vi "Z6_Beamline_Chief.ProcCases.vi"(0 "i ref in":refnum<vi>, 1 "selector":string, 2 "Data":T1, 3 "call cluster":T2={"Object"="", "Selector"="", "CallType"=enum."synchronous", "Async Object"="", "Async Selector"="", "Data Descriptor"="", "Data"=[], "Error #"=0, "Expire"=0}, 5 "error in (no error)":errorcluster) -> (14 "i ref out":refnum<vi>, 17 "answer cluster":T2={"Object"="", "Selector"="", "CallType"=enum."synchronous", "Async Object"="", "Async Selector"="", "Data Descriptor"="", "Data"=[], "Error #"=0, "Expire"=0}, 19 "error out":errorcluster)   [LabVIEW 2014, in "Z6_Beamline_Chief.lvlib"]
doc: "This method is called by a process from within the default case in the event loop. The methods of a class that are linked to events will be called from THIS method. Add your code here."
uses:
  Z6_Beamline_Chief.lvlib
  CSCore/CSSystem/CoreDefs/CoreDefs.call_type.ctl
  CSCore/BaseProcess/BaseProcess.descriptor string definition.ctl
  CSCore/CSSystem/CoreDefs/CoreDefs.rawDataType.ctl
  PH_BL-Master/PH_BL-Master.lvlib
  Z6_Beamline/Z6_Beamline.lvlib
  CSCore/BaseProcess/BaseProcess.lvlib
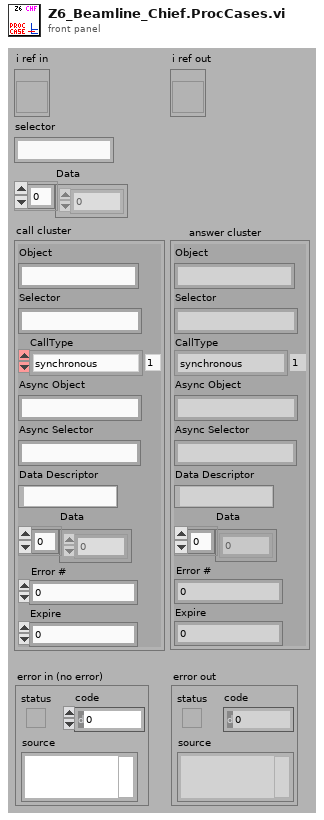
[diagram p1: front panel]
types:
  T1 = typedef "CoreDefs.rawDataType.ctl" = i8[]
  T2 = typedef "CoreDefs.call_type.ctl" = cluster{"Object":string, "Selector":string, "CallType":enum16{"simple", "synchronous", "asynchronous"}, "Async Object":string, "Async Selector":string, "Data Descriptor":T3, "Data":T1, "Error #":i32, "Expire":u32}
  T3 = typedef "BaseProcess.lvlib/BaseProcess.descriptor string definition.ctl" = string
  T4 = typedef "PH_BL-Master.lvlib/PH_BL-Master.i attribute.ctl" = cluster{"Remote controlled":bool, "Boolean Condition Service Subscriber":refnum<vi>[], "Picture Condition Service Subscriber":refnum<vi>[], "R2S":cluster{"GUI Ref":refnum<vi>, "State":bool}, "Vacua":cluster{"GUI Ref":refnum<vi>, "Limit":dbl, "Curr Value":dbl, "in range":bool}[], "O2 Inspection":cluster{"GUI Ref":refnum<vi>, "Concentration":dbl, "State":T5}[], "Boolean Status Service Subscriber":cluster{"GUI Ref":refnum<vi>, "Status":T5, "no Link?":bool, "Status Subscriber Class":T6}[], "Picture Status Service Subscriber":cluster{"GUI Ref":refnum<vi>, "Status":T5, "no Link?":bool, "Status Subscriber Class":T6}[], "6P 4Q Service Subscriber":cluster{"GUI Ref":refnum<vi>, "Selector":T7, "no Link?":bool}[], "Index of latest 6P 4Q changing Instance":i32, "Index of latest Picture Status changing Instance":i32, "Index of latest Boolean Status changing Instance":i32, "Vision ID on same Node":string, "Start Phase over?":bool, "GUI Ref Delete":refnum<vi>}
  T5 = typedef "PH_StatusHandler.lvlib/PH_StatusHandler.Status.ctl" = i16
  T6 = typedef "PH_BL-Master.lvlib/PH_BL-Master.Status Subscriber Class.ctl" = enum16{"unknown", "Switch", "BB", "6P Switch", "Switch GUI", "Switch and 6P State", "Force Sensor"}
  T7 = typedef "PH_4_Pos_Selector.lvlib/PH_4_Pos_Selector.Position Selector.ctl" = u16
  T8 = cluster{"GUI Ref":refnum<vi>, "Status":T5, "no Link?":bool, "Status Subscriber Class":T6}[]
  T9 = cluster{"GUI Ref":refnum<vi>, "Limit":dbl, "Curr Value":dbl, "in range":bool}[]
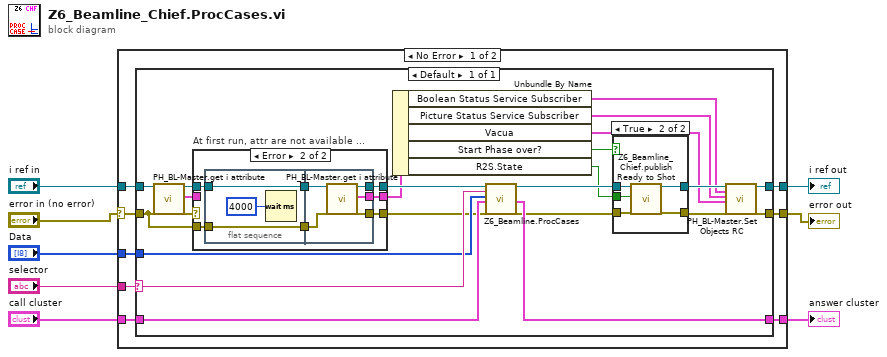
[diagram p0: block diagram]
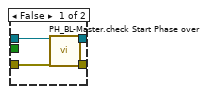
[diagram p3: hidden frame]
diagram:
  n1 = case shown="No Error" "error in (no error)" {
    selector: "error in (no error)" -> [w9 w68]
    tunnel: "selector" -> [w16 _]
    tunnel: [w15 w67] -> w7
    tunnel: "call cluster" -> [w14 w67]
    tunnel: "i ref in" -> [w13 w69]
    tunnel: [w12 w69] -> w4
    tunnel: [w11 w68] -> w3
    tunnel: "Data" -> [w10 _]
    frame No Error {
      n2 = case shown="Default" w16 {
        selector: w16 -> [w37]
        tunnel: w13 -> [w22]
        tunnel: [w33] -> w12
        tunnel: w14 -> [w38]
        tunnel: [w39] -> w15
        tunnel: w9 -> [w20]
        tunnel: [w32] -> w11
        tunnel: w10 -> [w36]
        frame Default {
          n3 = call "PH_BL-Master.get i attribute.vi"("i ref in"=w22, "error in (no error)"=w20) -> ("i ref out"=w21:refnum<vi>, "i attribute"=w18:T4, "error out"=w19:errorcluster)  [unwired: 15 in]
          n4 = case "At first run, attr are not available ..." shown="Error" w19 {
            selector: w19 -> [w41 _]
            tunnel: [w41 w49] -> w31
            tunnel: [w42 w48] -> w30
            tunnel: [w40 w47] -> w27
            tunnel: w21 -> [w42 w46]
            tunnel: w20 -> [_ w45]
            tunnel: w18 -> [w40 _]
            frame No Error {
            }
            frame Error {
              n5 = flat-sequence {
                tunnel: w45 -> [w51]
                tunnel: w46 -> [w52]
                tunnel: [w52] -> w44
                tunnel: [w51] -> w43
                tunnel: [w57] -> w49
                tunnel: [w56] -> w48
                tunnel: [w55] -> w47
                tunnel: w44 -> [w54]
                tunnel: w43 -> [w53]
                frame #0 {
                  n6 = Wait (ms)(milliseconds to wait=u32 4000) -> ()  [unwired: 1 out]
                }
                frame #1 {
                  n7 = call "PH_BL-Master.get i attribute.vi"("i ref in"=w54, "error in (no error)"=w53) -> ("i ref out"=w56:refnum<vi>, "i attribute"=w55:T4, "error out"=w57:errorcluster)  [unwired: 15 in]
                }
              }
            }
          }
          n8 = Unbundle By Name(w27) -> ("Boolean Status Service Subscriber"=w23:T8, "Picture Status Service Subscriber"=w24:T8, "Vacua"=w25:T9, "Start Phase over?"=w26:bool, "R2S.State"=w17:bool)
          n9 = call "Z6_Beamline.ProcCases.vi"("i ref in"=w30, "selector"=w37, "Data"=w36, "call cluster"=w38, "error in (no error)"=w31) -> ("i ref out"=w28:refnum<vi>, "answer cluster"=w39:T2, "error out"=w29:errorcluster)  [unwired: 12 in]
          n10 = case shown="True" w26 {
            tunnel: [w60 w64] -> w34
            tunnel: [w58 w63] -> w35
            tunnel: w29 -> [w59 w66]
            tunnel: w28 -> [w61 w65]
            tunnel: w17 -> [_ w62]
            frame False {
              n11 = call "PH_BL-Master.check Start Phase over.vi"("VI in"=w61, "error in (no error)"=w59) -> ("VI out"=w60:refnum<vi>, "error out"=w58:errorcluster)  [unwired: 16 in]
            }
            frame True {
              n12 = call "Z6_Beamline_Chief.publish Ready to Shot.vi"("i ref in"=w65, "R2S before"=w62, "error in (no error)"=w66) -> ("i ref out"=w64:refnum<vi>, "error out"=w63:errorcluster)  [unwired: 15 in]
            }
          }
          n13 = call "PH_BL-Master.Set Objects RC.vi"("VI in"=w34, "Boolean Status Service Subscriber before"=w23, "Picture Status Service Subscriber before"=w24, "Vacua before"=w25, "error in (no error)"=w35) -> ("VI out"=w33:refnum<vi>, "error out"=w32:errorcluster)  [unwired: 13 in]
        }
      }
    }
    frame Error {
    }
  }
  "answer cluster" <- w7
  "i ref out" <- w4
  "error out" <- w3
